vi "Image FGV.vi"(7 "Image action":T3, 8 "error in (no error)":errorcluster, 9 "Image Type":T1 items=["Grayscale (U8)", "Grayscale (I16)", "Grayscale (SGL)", "Complex (CSG)", "RGB (U32)", "HSL (U32)", "RGB (U64)", "Grayscale (U16)"], 10 "Image In":T2, 11 "圖片名稱":string) -> (0 "error out":errorcluster, 2 "Image Out":T2)   [LabVIEW 2015]
uses:
  Control/Image action.ctl
  <vilib>/vision/Image Controls.llb/IMAQ Image.ctl
  <vilib>/vision/NI_Vision_Development_Module.lvlib
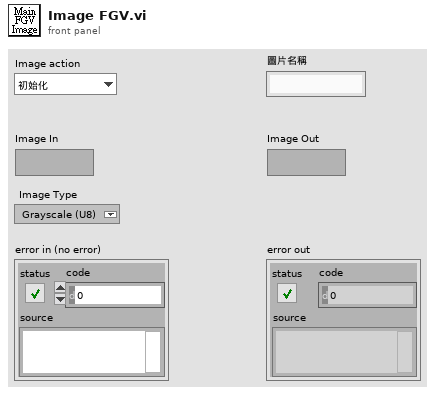
[diagram p1: front panel]
types:
  T1 = typedef "Image Type" = u32
  T2 = typedef "IMAQ Image.ctl" = refnum<image>
  T3 = typedef "Image action.ctl" = enum16{"初始化", "創造記憶體", "寫入圖片", "讀取圖片", "刪除圖片", "等待"}
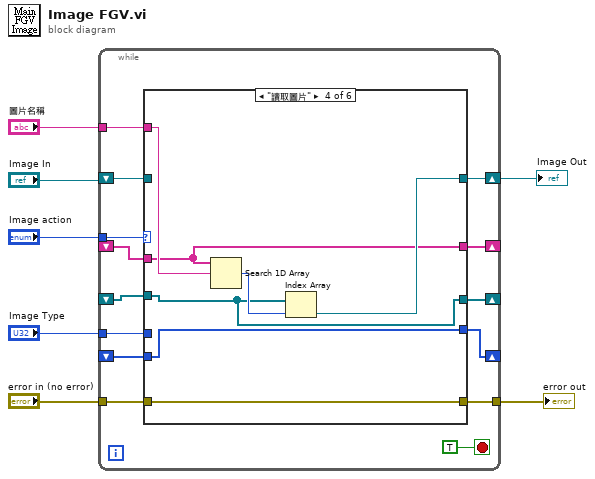
[diagram p0: block diagram]
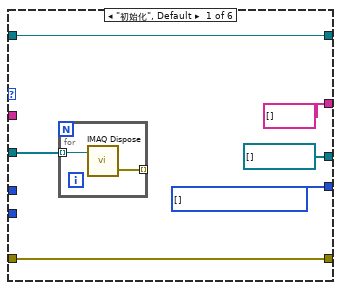
[diagram p2: hidden frame]
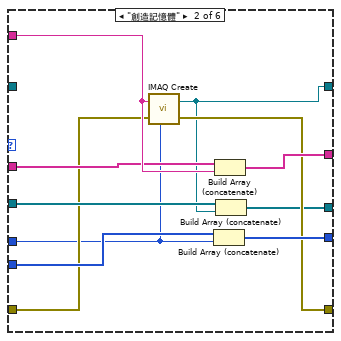
[diagram p3: hidden frame]
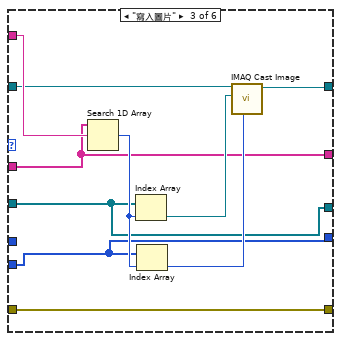
[diagram p4: hidden frame]
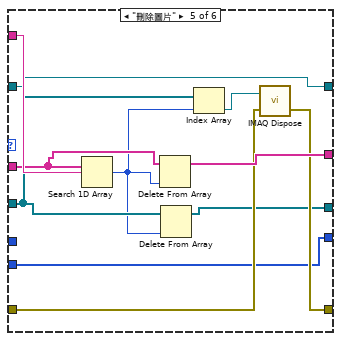
[diagram p5: hidden frame]
diagram:
  n1 = while {
    tunnel: "Image action" -> [w20]
    tunnel: "圖片名稱" -> [w19]
    shift-right: [w18] -> _
    shift-left: _ -> [w16]
    shift-right: [w8] -> w1
    shift-left: "Image In" -> [w17]
    shift-right: [w15] -> _
    shift-left: _ -> [w14]
    shift-right: [w12] -> _
    shift-left: _ -> [w11]
    tunnel: "Image Type" -> [w13]
    tunnel: "error in (no error)" -> [w10]
    tunnel: [w9] -> w2
    stop <- TRUE stop-if-true
    n2 = case shown="\"讀取圖片\"" w20 {
      tunnel: w19 -> [_ w40 w50 w57 w68 _]
      tunnel: [string[] [] w39 w41 w51 w66 w72] -> w18
      tunnel: w17 -> [w22 _ w45 _ w58 w73]
      tunnel: w16 -> [_ w38 w41 w51 w67 w72]
      tunnel: [T2[] [] w32 w42 w52 w59 w71] -> w15
      tunnel: w14 -> [w27 w37 w42 w52 w61 w71]
      tunnel: w13 -> [_ w31 _ _ _ _]
      tunnel: [w25 w36 w43 w53 w62 w70] -> w12
      tunnel: w11 -> [_ w35 w43 w53 w62 w70]
      tunnel: w10 -> [w26 w34 w44 w54 w63 w69]
      tunnel: [w26 w33 w44 w54 w65 w69] -> w9
      tunnel: [w22 w30 w48 w55 w58 w73] -> w8
      frame "初始化", Default {
        w25 = T1[] [] items=["Grayscale (U8)", "Grayscale (I16)", "Grayscale (SGL)", "Complex (CSG)", "RGB (U32)", "HSL (U32)", "RGB (U64)", "Grayscale (U16)"]
        n3 = for {
          tunnel: w27 -> [w29] mode=indexing
          tunnel: [w28] -> _ mode=indexing
          n4 = call "IMAQ Dispose"("Image"=w29) -> ("error out"=w28:errorcluster)  [unwired: 5 in]
        }
      }
      frame "創造記憶體" {
        n5 = call "IMAQ Create"("Image Name"=w40, "Image Type"=w31, "error in (no error)"=w34) -> ("New Image"=w30:T2, "error out"=w33:errorcluster)  [unwired: 2 in]
        n6 = Build Array (concatenate)(w35, w31) -> (w36:T1[])
        n7 = Build Array (concatenate)(w38, w40) -> (w39:string[])
        n8 = Build Array (concatenate)(w37, w30) -> (w32:T2[])
      }
      frame "寫入圖片" {
        n9 = Search 1D Array(1D array=w41, element=w50) -> (index of element=w49:i32)  [unwired: 1 in]
        n10 = Index Array(array=w42, index=w49) -> (element=w46:T2)
        n11 = Index Array(array=w43, index=w49) -> (element=w47:T1)
        n12 = call "IMAQ Cast Image"("Image Type"=w47, "Image Dst"=w46, "Image Src"=w45) -> ("Image Dst Out"=w48:T2)  [unwired: 7 in, 1 out]
      }
      frame "讀取圖片" {
        n13 = Search 1D Array(1D array=w51, element=w57) -> (index of element=w56:i32)  [unwired: 1 in]
        n14 = Index Array(array=w52, index=w56) -> (element=w55:T2)
      }
      frame "刪除圖片" {
        n15 = Search 1D Array(1D array=w67, element=w68) -> (index of element=w60:i32)  [unwired: 1 in]
        n16 = Delete From Array(array=w67, index=w60) -> (array with subset deleted=w66:string[])  [unwired: 1 in, 1 out]
        n17 = Delete From Array(array=w61, index=w60) -> (array with subset deleted=w59:T2[])  [unwired: 1 in, 1 out]
        n18 = Index Array(array=w61, index=w60) -> (element=w64:T2)
        n19 = call "IMAQ Dispose"("Image"=w64, "error in (no error)"=w63) -> ("error out"=w65:errorcluster)  [unwired: 4 in]
      }
      frame "等待" {
      }
    }
  }
  "error out" <- w2
  "Image Out" <- w1
